vi "close.vi"(2 "error in":errorcluster) -> (0 "error out":errorcluster)   [LabVIEW 2016, in "labssh_thijs.lvlib"]
uses:
  labssh_thijs.lvlib
  Labview SSH driver/state machine.ctl
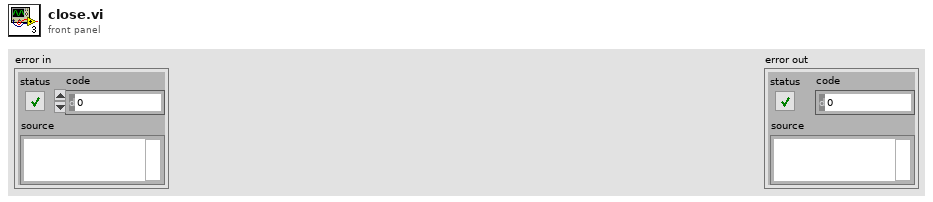
[diagram p1: front panel]
types:
  T1 = typedef "labssh_thijs.lvlib/state machine.ctl" = enum16{"init", "connect", "execute", "close", "exit", "read"}
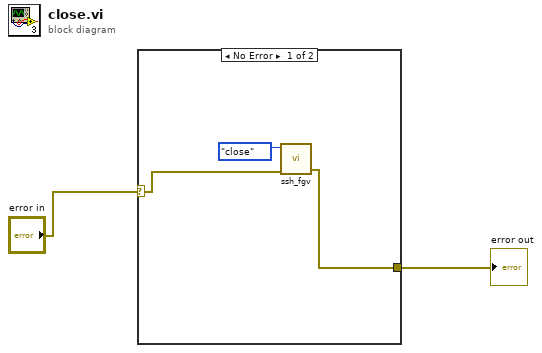
[diagram p0: block diagram]
diagram:
  n1 = case shown="No Error" "error in" {
    selector: "error in" -> [w4 w6]
    tunnel: [w3 w6] -> w1
    frame No Error {
      n2 = call "ssh_fgv.vi"(0:state_machine."close", "error in"=w4) -> ("error out"=w3:errorcluster)  [unwired: 5 in, 1 out]
    }
    frame Error {
    }
  }
  "error out" <- w1
